vi "PI acquire semaphore.vi"(0 "System no.":i32=1 min=1 step=1, 5 "error in":errorcluster) -> (14 "timed out":bool, 15 "semaphore out":T1, 19 "error out":errorcluster)   [LabVIEW 2026]
doc: "This VI acquires the semaphore that was defined in Global1.vi for the specified system during initialization."
uses:
  Global1.vi
panel:
  # "This vi acquires the semaphore that was defined in Global1.vi for the specified system."
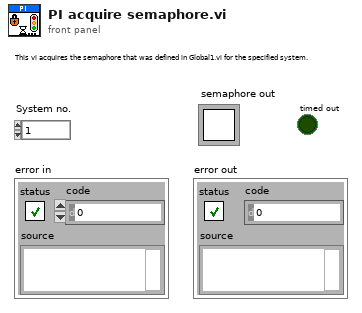
[diagram p1: front panel]
types:
  T1 = typedef "Semaphore RefNum" = refnum<k1>
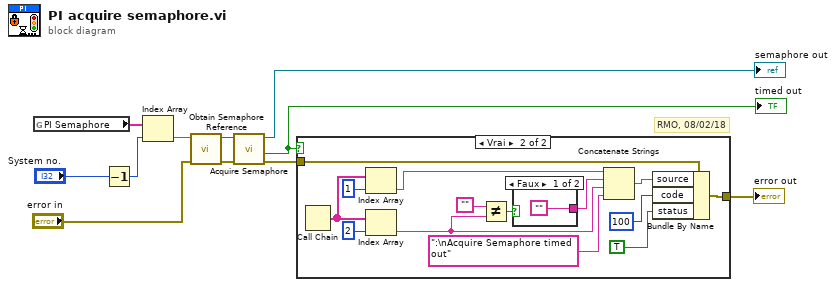
[diagram p0: block diagram]
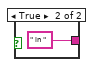
[diagram p3: hidden frame]
diagram:
  # "RMO, 08/02/18"
  n1 = global read "Global1.vi" "PI Semaphore"() -> (w6:string[])
  n2 = Decrement(x="System no.") -> (x-1=w5:i32)
  n3 = Index Array(array=w6, index=w5) -> (element=w2:string)
  n4 = call <vilib>:"Obtain Semaphore Reference.vi"("error in (no error)"="error in", "name (unnamed)"=w2) -> ("error out"=w4:errorcluster, "semaphore"=w3:T1)  [unwired: 1 in, 3 out]
  n5 = call <vilib>:"Acquire Semaphore.vi"("error in (no error)"=w4, "semaphore"=w3) -> ("error out"=w7:errorcluster, "timed out"=w10:bool, "semaphore out"=→"semaphore out":T1)  [unwired: 1 in, 2 out]
  "timed out" <- w10
  n6 = case shown="Vrai" w10 {
    tunnel: w7 -> [w12 w25]
    tunnel: [w12 w23] -> w11
    frame False {
    }
    frame True {
      n7 = Call Chain() -> (call chain=w14:string[])
      n8 = Index Array(array=w14, index=1) -> (element=w13:string)
      n9 = Index Array(array=w14, index=2) -> (element=w19:string)
      n10 = Not Equal?(x="", y=w19) -> (x != y?=w17:bool)
      n11 = case shown="Faux" w17 {
        tunnel: ["" " in " ("source")] -> w16
        frame False {
        }
        frame True {
        }
      }
      n12 = Concatenate Strings(w13, w16, w19, ":\nAcquire Semaphore timed out" ("source")) -> (w22:string)
      n13 = Bundle By Name(cluster=w25, "source"=w22, "code"=100 ("index"), "status"=TRUE) -> (w23:errorcluster)
    }
  }
  "error out" <- w11
